vi "Joint Reference Follower v1.3.vi"(6 "Accurus Ctrl Cluster":T2={"Stop Vacuum"=TRUE, "Vacuum Force"=0, "Max Limit [mmHg]"=600.0, "Slide in"=0, "Irrigation?"=TRUE} {"Slide in" scale=0.0..78.0; "Vacuum Force" min=0 max=78}, 7 "Offset Home2RCM [deg/mm]":dbl[](array[numeric])=[0.0, 0.0, 0.0, 0.0], 8 "PID Ctrl Cluster":T3={"L1 PID Gains"={"Kp"=0.005, "Kd"=0.5, "Ki"=0.0005}, "L2 PID Gains"={"Kp"=0.01, "Kd"=1.0, "Ki"=0.005}, "L3 PID Gains"={"Kp"=0.05, "Kd"=1.0, "Ki"=0.0005}, "L4 PID Gains"={"Kp"=0.1, "Kd"=0.1, "Ki"=0.0005}}, 9 "Ref Array [deg/mm]":dbl[](array[numeric])=[0.0, 0.0, 0.0, 0.0], 10 "error in":errorcluster, 11 "FPGA VI Reference In":refnum<k20>) -> (0 "Accurus Output Cluster":T1, 1 "Output Posit Array [deg/mm]":dbl[](array[numeric]), 2 "error out":errorcluster, 3 "FPGA VI Reference Out":refnum<k20>)   [LabVIEW 2010]
uses:
  <vilib>/rvi/interface/nirviReadWriteControl/nirviReadWriteControl.xnode
  Library/KevinLibraryAll/labview/KevLib01.lvlib
  Subsystems/Global Variables.vi
  FPGA Bitfiles/IRISSControl_FPGATarget_IRISSFPGAIOv3.3_r-h2UkgnQFc.lvbitx
  IRISS_FPGA_IO_v3.3.vi
panel:
  # "button 1"
  # "button 2"
  # "button 3"
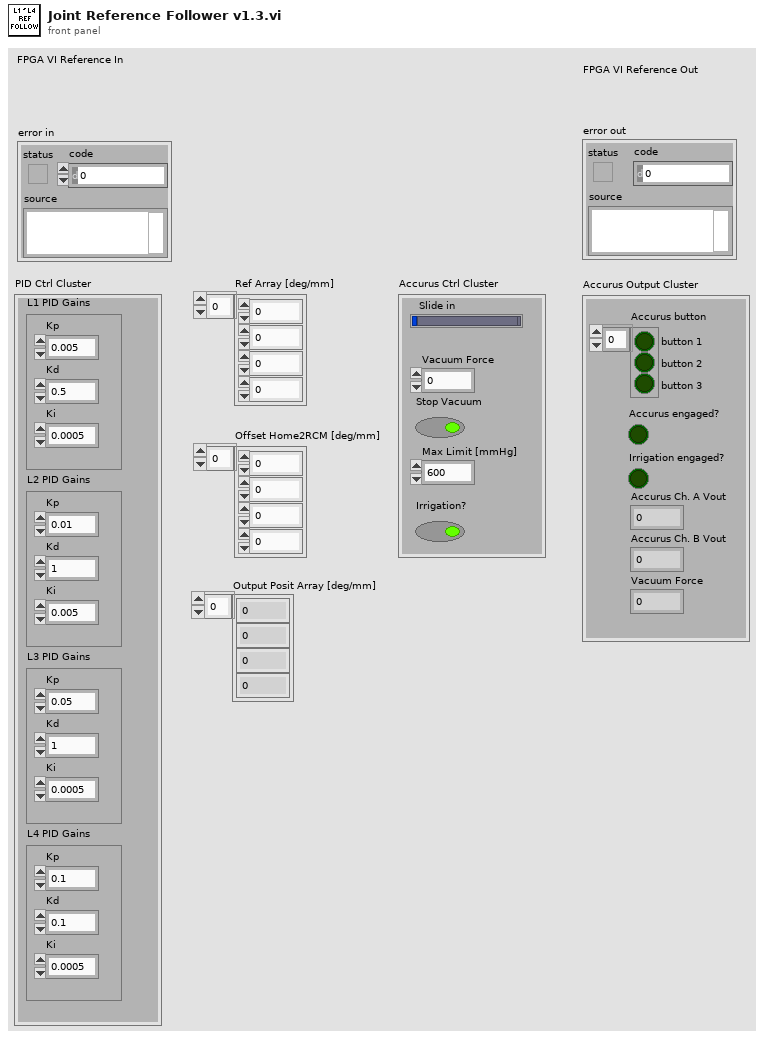
[diagram p1: front panel]
types:
  T1 = cluster{"Accurus button":bool[], "Accurus engaged?":bool, "Vacuum Force":i32, "Accurus Ch. A Vout":dbl, "Accurus Ch. B Vout":dbl, "Irrigation engaged?":bool}
  T2 = cluster{"Stop Vacuum":bool, "Vacuum Force":i8, "Max Limit [mmHg]":dbl, "Slide in":i8, "Irrigation?":bool}
  T3 = cluster{"L1 PID Gains":cluster{"Kp":dbl, "Kd":dbl, "Ki":dbl}, "L2 PID Gains":cluster{"Kp":dbl, "Kd":dbl, "Ki":dbl}, "L3 PID Gains":cluster{"Kp":dbl, "Kd":dbl, "Ki":dbl}, "L4 PID Gains":cluster{"Kp":dbl, "Kd":dbl, "Ki":dbl}}
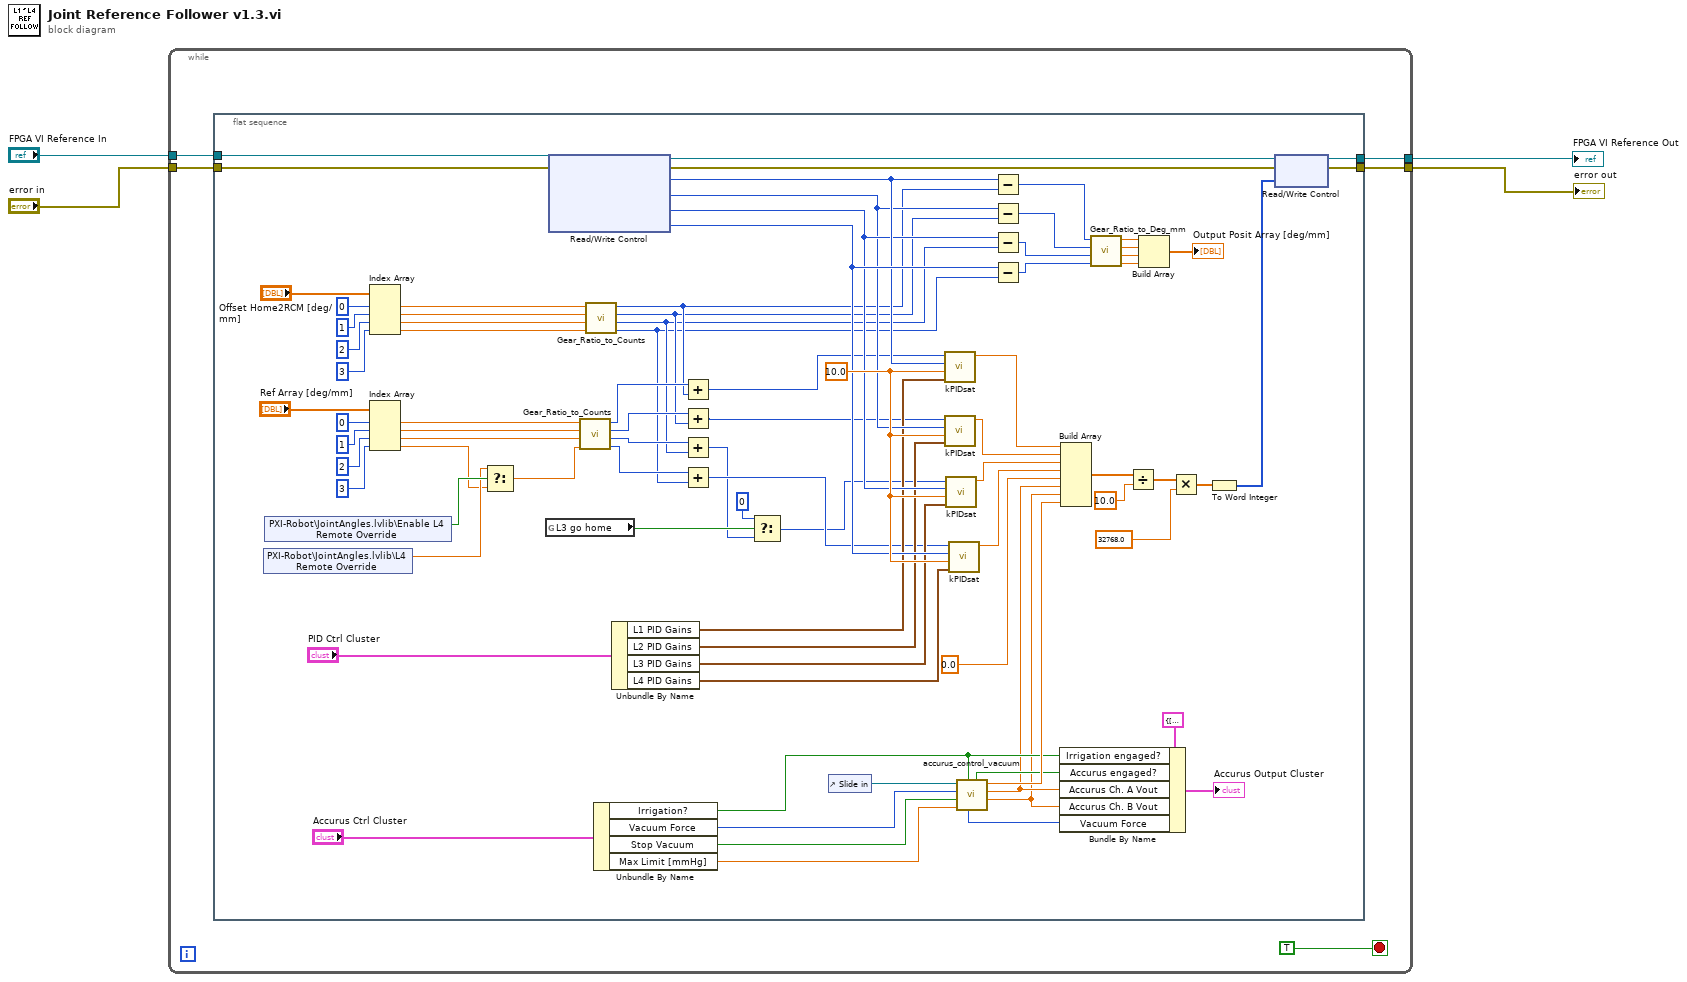
[diagram p0: block diagram]
diagram:
  n1 = while {
    tunnel: [w9] -> w4
    tunnel: [w8] -> w3
    tunnel: "FPGA VI Reference In" -> [w7]
    tunnel: "error in" -> [w6]
    stop <- TRUE ("Boolean") stop-if-true
    n2 = flat-sequence {
      tunnel: [w70] -> w9
      tunnel: [w69] -> w8
      tunnel: w7 -> [w46]
      tunnel: w6 -> [w45]
      frame #0 {
        w80 = 10.0 ("Sat Limit")
        n3 = shared-variable "PXI-Robot\\JointAngles.lvlib\\L4 Remote Override"() -> (w19:dbl)  [unwired: 1 in, 1 out]
        n4 = shared-variable "PXI-Robot\\JointAngles.lvlib\\Enable L4 Remote Override"() -> (w20:bool)  [unwired: 1 in, 1 out]
        n5 = Index Array(array="Offset Home2RCM [deg/mm]", index #1=0 ("index"), index #2=1 ("index"), index #3=2 ("index"), index #4=3 ("index")) -> (element #1=w44:dbl, element #2=w43:dbl, element #3=w42:dbl, element #4=w41:dbl)
        n6 = Index Array(array="Ref Array [deg/mm]", index #1=0 ("index"), index #2=1 ("index"), index #3=2 ("index"), index #4=3 ("index")) -> (element #1=w88:dbl, element #2=w87:dbl, element #3=w86:dbl, element #4=w18:dbl)
        n7 = Select(t=w19, s=w20, f=w18) -> (s? t:f=w17:dbl)
        n8 = global read "Global Variables.vi" "L3 go home"() -> (w24:bool)
        n9 = xnode "Read/Write Control"("FPGA VI Reference In"=w46, "error in"=w45) -> ("FPGA VI Reference Out"=w72:refnum<k20>, "error out"=w71:errorcluster, "32 bit Position 1"=w53:i32, "32 bit Position 3"=w51:i32, "32 bit Position C1-1"=w52:i32, "32 bit Position C1-4"=w63:i32)
        n10 = call "Gear_Ratio_to_Counts.vi"("theta 4"=w17, "theta 3"=w86, "theta 2"=w87, "theta 1"=w88) -> ("j4"=w34:i32, "j3"=w35:i32, "j2"=w36:i32, "j1"=w37:i32)
        n11 = call "Gear_Ratio_to_Counts.vi"("theta 4"=w41, "theta 3"=w42, "theta 2"=w43, "theta 1"=w44) -> ("j4"=w30:i32, "j3"=w31:i32, "j2"=w32:i32, "j1"=w33:i32)
        n12 = Unbundle By Name("Accurus Ctrl Cluster") -> ("Irrigation?"=w15:bool, "Vacuum Force"=w28:i8, "Stop Vacuum"=w27:bool, "Max Limit [mmHg]"=w26:dbl)
        n13 = Unbundle By Name("PID Ctrl Cluster") -> ("L1 PID Gains"=w50:cluster{"Kp":dbl, "Kd":dbl, "Ki":dbl}, "L2 PID Gains"=w49:cluster{"Kp":dbl, "Kd":dbl, "Ki":dbl}, "L3 PID Gains"=w48:cluster{"Kp":dbl, "Kd":dbl, "Ki":dbl}, "L4 PID Gains"=w47:cluster{"Kp":dbl, "Kd":dbl, "Ki":dbl})
        n14 = Add(x=w37, y=w33) -> (x+y=w40:i32)
        n15 = Add(x=w36, y=w32) -> (x+y=w39:i32)
        n16 = Add(x=w35, y=w31) -> (x+y=w23:i32)
        n17 = Add(x=w34, y=w30) -> (x+y=w38:i32)
        n18 = Select(t=0 ("index"), s=w24, f=w23) -> (s? t:f=w21:i32)
        n19 = control-ref of="Slide in"() -> (w25:refnum<vi>)
        n20 = call "kPIDsat.vi"("PID Gains"=w50, "Sat Limit"=w80, "Position"=w53, "Reference"=w40) -> ("Control"=w62:dbl)  [unwired: 7 in]
        n21 = call "kPIDsat.vi"("PID Gains"=w49, "Sat Limit"=w80, "Position"=w51, "Reference"=w39) -> ("Control"=w64:dbl)  [unwired: 7 in]
        n22 = call "kPIDsat.vi"("PID Gains"=w48, "Sat Limit"=w80, "Position"=w52, "Reference"=w21) -> ("Control"=w65:dbl)  [unwired: 7 in]
        n23 = call "kPIDsat.vi"("PID Gains"=w47, "Sat Limit"=w80, "Position"=w63, "Reference"=w38) -> ("Control"=w79:dbl)  [unwired: 7 in]
        n24 = call "accurus_control_vacuum.vi"("Irrigate?"=w15, "Max Limit [mmHg]"=w26, "stop"=w27, "vacuum force"=w28, "Slide in"=w25) -> ("f"=w12:dbl, "f 2"=w13:dbl, "f 3"=w67:dbl, "Boolean 2"=w14:bool, "Vacuum Force\n[mmHg]"=w11:i32)  [unwired: 1 in, 1 out]
        n25 = Subtract(x=w53, y=w33) -> (x-y=w57:i32)
        n26 = Subtract(x=w51, y=w32) -> (x-y=w56:i32)
        n27 = Subtract(x=w52, y=w31) -> (x-y=w55:i32)
        n28 = Subtract(x=w63, y=w30) -> (x-y=w54:i32)
        n29 = Bundle By Name(cluster=T1 {"Accurus button"=[FALSE, FALSE, FALSE], "Accurus engaged?"=FALSE, "Vacuum Force"=0, "Accurus Ch. A Vout"=0.0, "Accurus Ch. B Vout"=0.0, "Irrigation engaged?"=FALSE} ("Accurus Output Cluster"), "Irrigation engaged?"=w15, "Accurus engaged?"=w14, "Accurus Ch. A Vout"=w13, "Accurus Ch. B Vout"=w12, "Vacuum Force"=w11) -> (→"Accurus Output Cluster":T1)
        n30 = Build Array(w62, w64, w65, w79, 0.0 ("element"), w13, w12, w67) -> (w78:dbl[])
        n31 = call "Gear_Ratio_to_Deg_mm.vi"("j4"=w54, "j3"=w55, "j2"=w56, "j1"=w57) -> ("theta 4"=w58:dbl, "theta 3"=w59:dbl, "theta 2"=w60:dbl, "theta 1"=w61:dbl)
        n32 = Divide(x=w78, y=10.0) -> (x/y=w76:dbl[])
        n33 = Build Array(w61, w60, w59, w58) -> (→"Output Posit Array [deg/mm]":dbl[])
        n34 = Multiply(x=w76, y=32768.0) -> (x*y=w74:dbl[])
        n35 = To Word Integer(number=w74) -> (16bit integer=w73:i16[])
        n36 = xnode "Read/Write Control"("FPGA VI Reference In"=w72, "error in"=w71, "AO"=w73) -> ("FPGA VI Reference Out"=w70:refnum<k20>, "error out"=w69:errorcluster)
      }
    }
  }
  "error out" <- w3
  "FPGA VI Reference Out" <- w4
